vi "test-discretization-14.vi"(8 "error in (no error)":errorcluster) -> (0 "error out":errorcluster, 3 "All Tests Passed":bool)   [LabVIEW 2019]
uses:
  <vilib>/Analysis/Matrix/Datatypes/ComplexMatrix.ctl
  <vilib>/Analysis/Matrix/Datatypes/RealMatrix.ctl
  <vilib>/Analysis/7linalg.llb/Eigenvalue and Vectors Output Option.ctl
  <vilib>/Rock Robotics/WPI/ThirdParty/JAS_Junk/TrajLib/MatBuilder_Create.vi
  <vilib>/Rock Robotics/WPI/ThirdParty/JAS_Junk/TrajLib/MatrixHelper_CoerceSize.vi
  <vilib>/Rock Robotics/WPI/ThirdParty/JAS_Junk/TrajLib/Matrix_Transpose.vi
  <vilib>/Rock Robotics/WPI/ThirdParty/JAS_Junk/TrajLib/Matrix_AssignBlock.vi
  <vilib>/Rock Robotics/WPI/ThirdParty/JAS_Junk/TrajLib/Matrix_Exp.vi
  <vilib>/Rock Robotics/WPI/ThirdParty/JAS_Junk/TrajLib/Matrix_Block.vi
  <vilib>/Analysis/baseanly.llb/A x B.vi
  <vilib>/Analysis/baseanly.llb/Real A x B.vi
  <vilib>/Analysis/7linalg.llb/Transpose Matrix.vi
  <vilib>/Analysis/7linalg.llb/Real Transpose Matrix.vi
  <vilib>/Analysis/_algsub.llb/Matrix Norm.vi
  <vilib>/Analysis/_algsub.llb/Real Matrix Norm.vi
  <vilib>/Analysis/7linalg.llb/Matrix Exp.vi
  <vilib>/Analysis/7linalg.llb/Real Matrix Exp.vi
  <vilib>/Analysis/7linalg.llb/Real Eigenvalues and Vectors.vi
  <vilib>/Analysis/Matrix/Numeric/Multiply/Multiply.vi
  <vilib>/Analysis/Matrix/Numeric/Multiply/Multiply - RM,R.vi
  <vilib>/Analysis/Matrix/Numeric/Add/Add.vi
  <vilib>/Analysis/Matrix/Numeric/Add/Add - RM,RM.vi
  <vilib>/Analysis/Matrix/Numeric/Subtract/Subtract - RM,RM.vi
  <vilib>/Rock Robotics/WPI/ThirdParty/JAS_Junk/TrajLib/Trajectory_Library.lvlib
  <vilib>/Analysis/NI_AALPro.lvlib
  <vilib>/Analysis/Matrix/NI_Matrix.lvlib
panel:
  out "Eigenvalues 2":cdb[](array[numeric])
  out "Pos Semidefiniate 2":bool
  out "error 2":i32
  out "ApproxEquals 2":bool
  out "ApproxEquals":bool
  out "DiscQ Taylor\nNOT":T1
  out "DiscA Taylor\nNOT":T1
  out "Error 2":bool
  out "DiscA":T1
  out "DiscQ Int":T1
  in  "Cluster":cluster{"ContQ":T1, "ContA":T1}
  out "int discq":bool
  out "Pos Semidefiniate":bool
  out "Eigenvectors":T2
  out "error":i32
  out "Eigenvalues":cdb[](array[numeric])
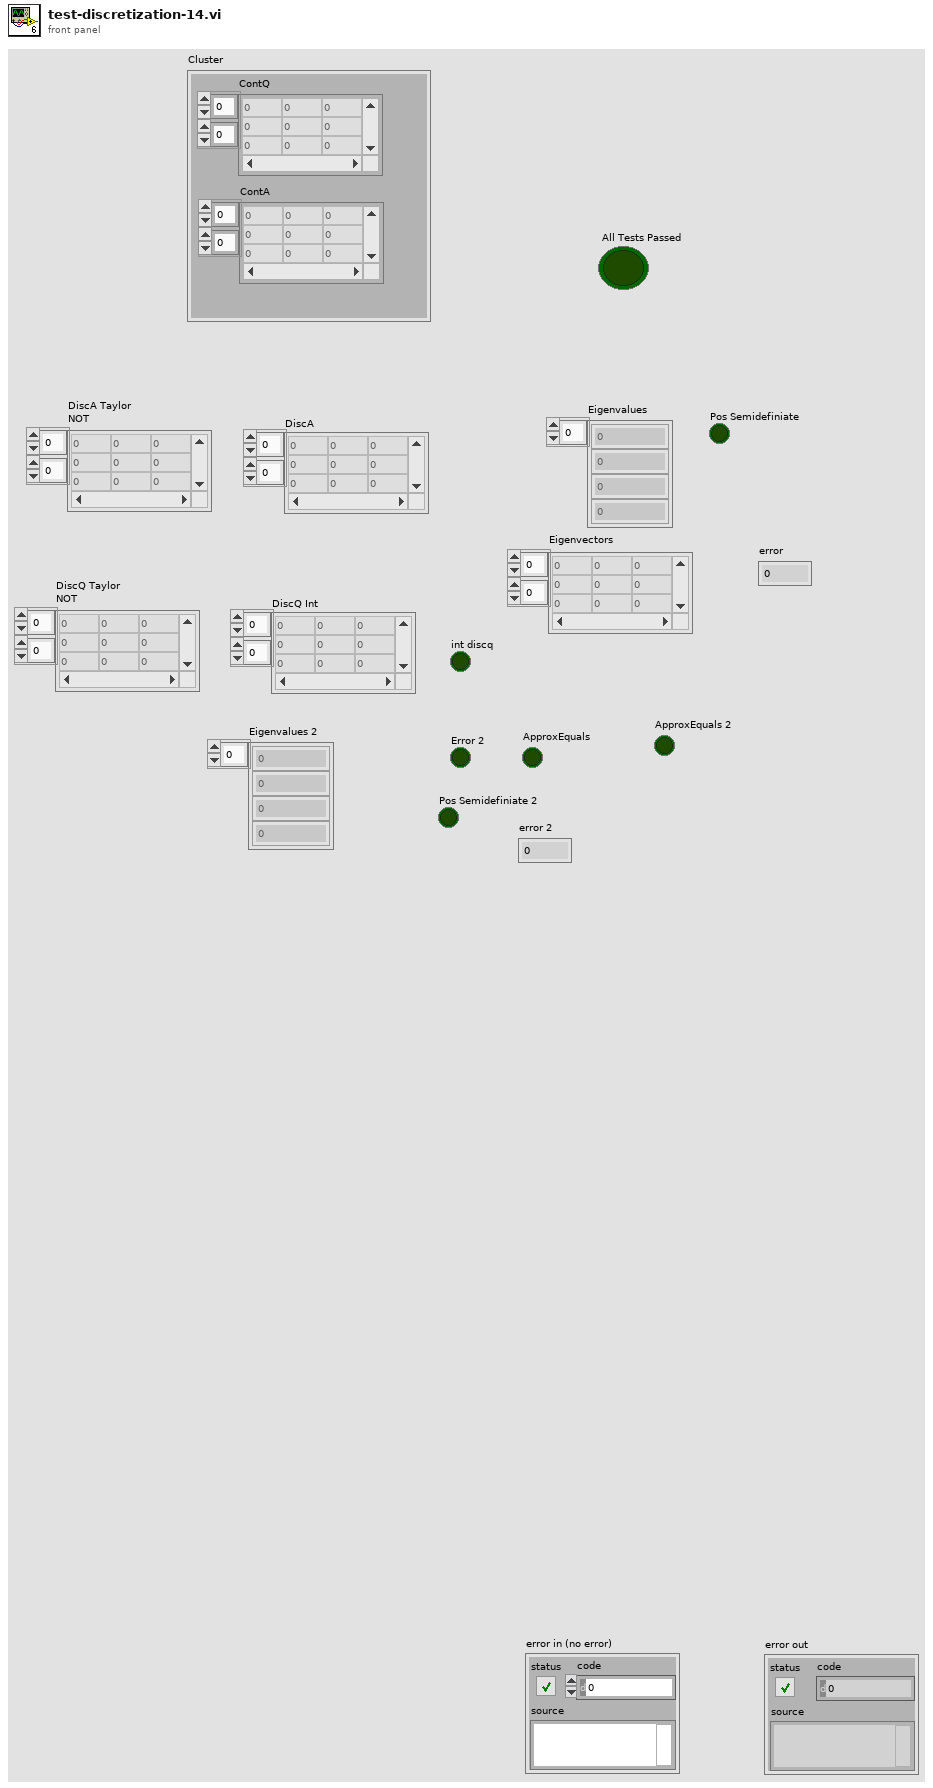
[diagram p1: front panel]
types:
  T1 = typedef "NI_Matrix.lvlib/RealMatrix.ctl" = dbl[][]
  T2 = typedef "NI_Matrix.lvlib/ComplexMatrix.ctl" = cdb[][]
  T3 = typedef "NI_AALPro.lvlib/Eigenvalue and Vectors Output Option.ctl" = i32
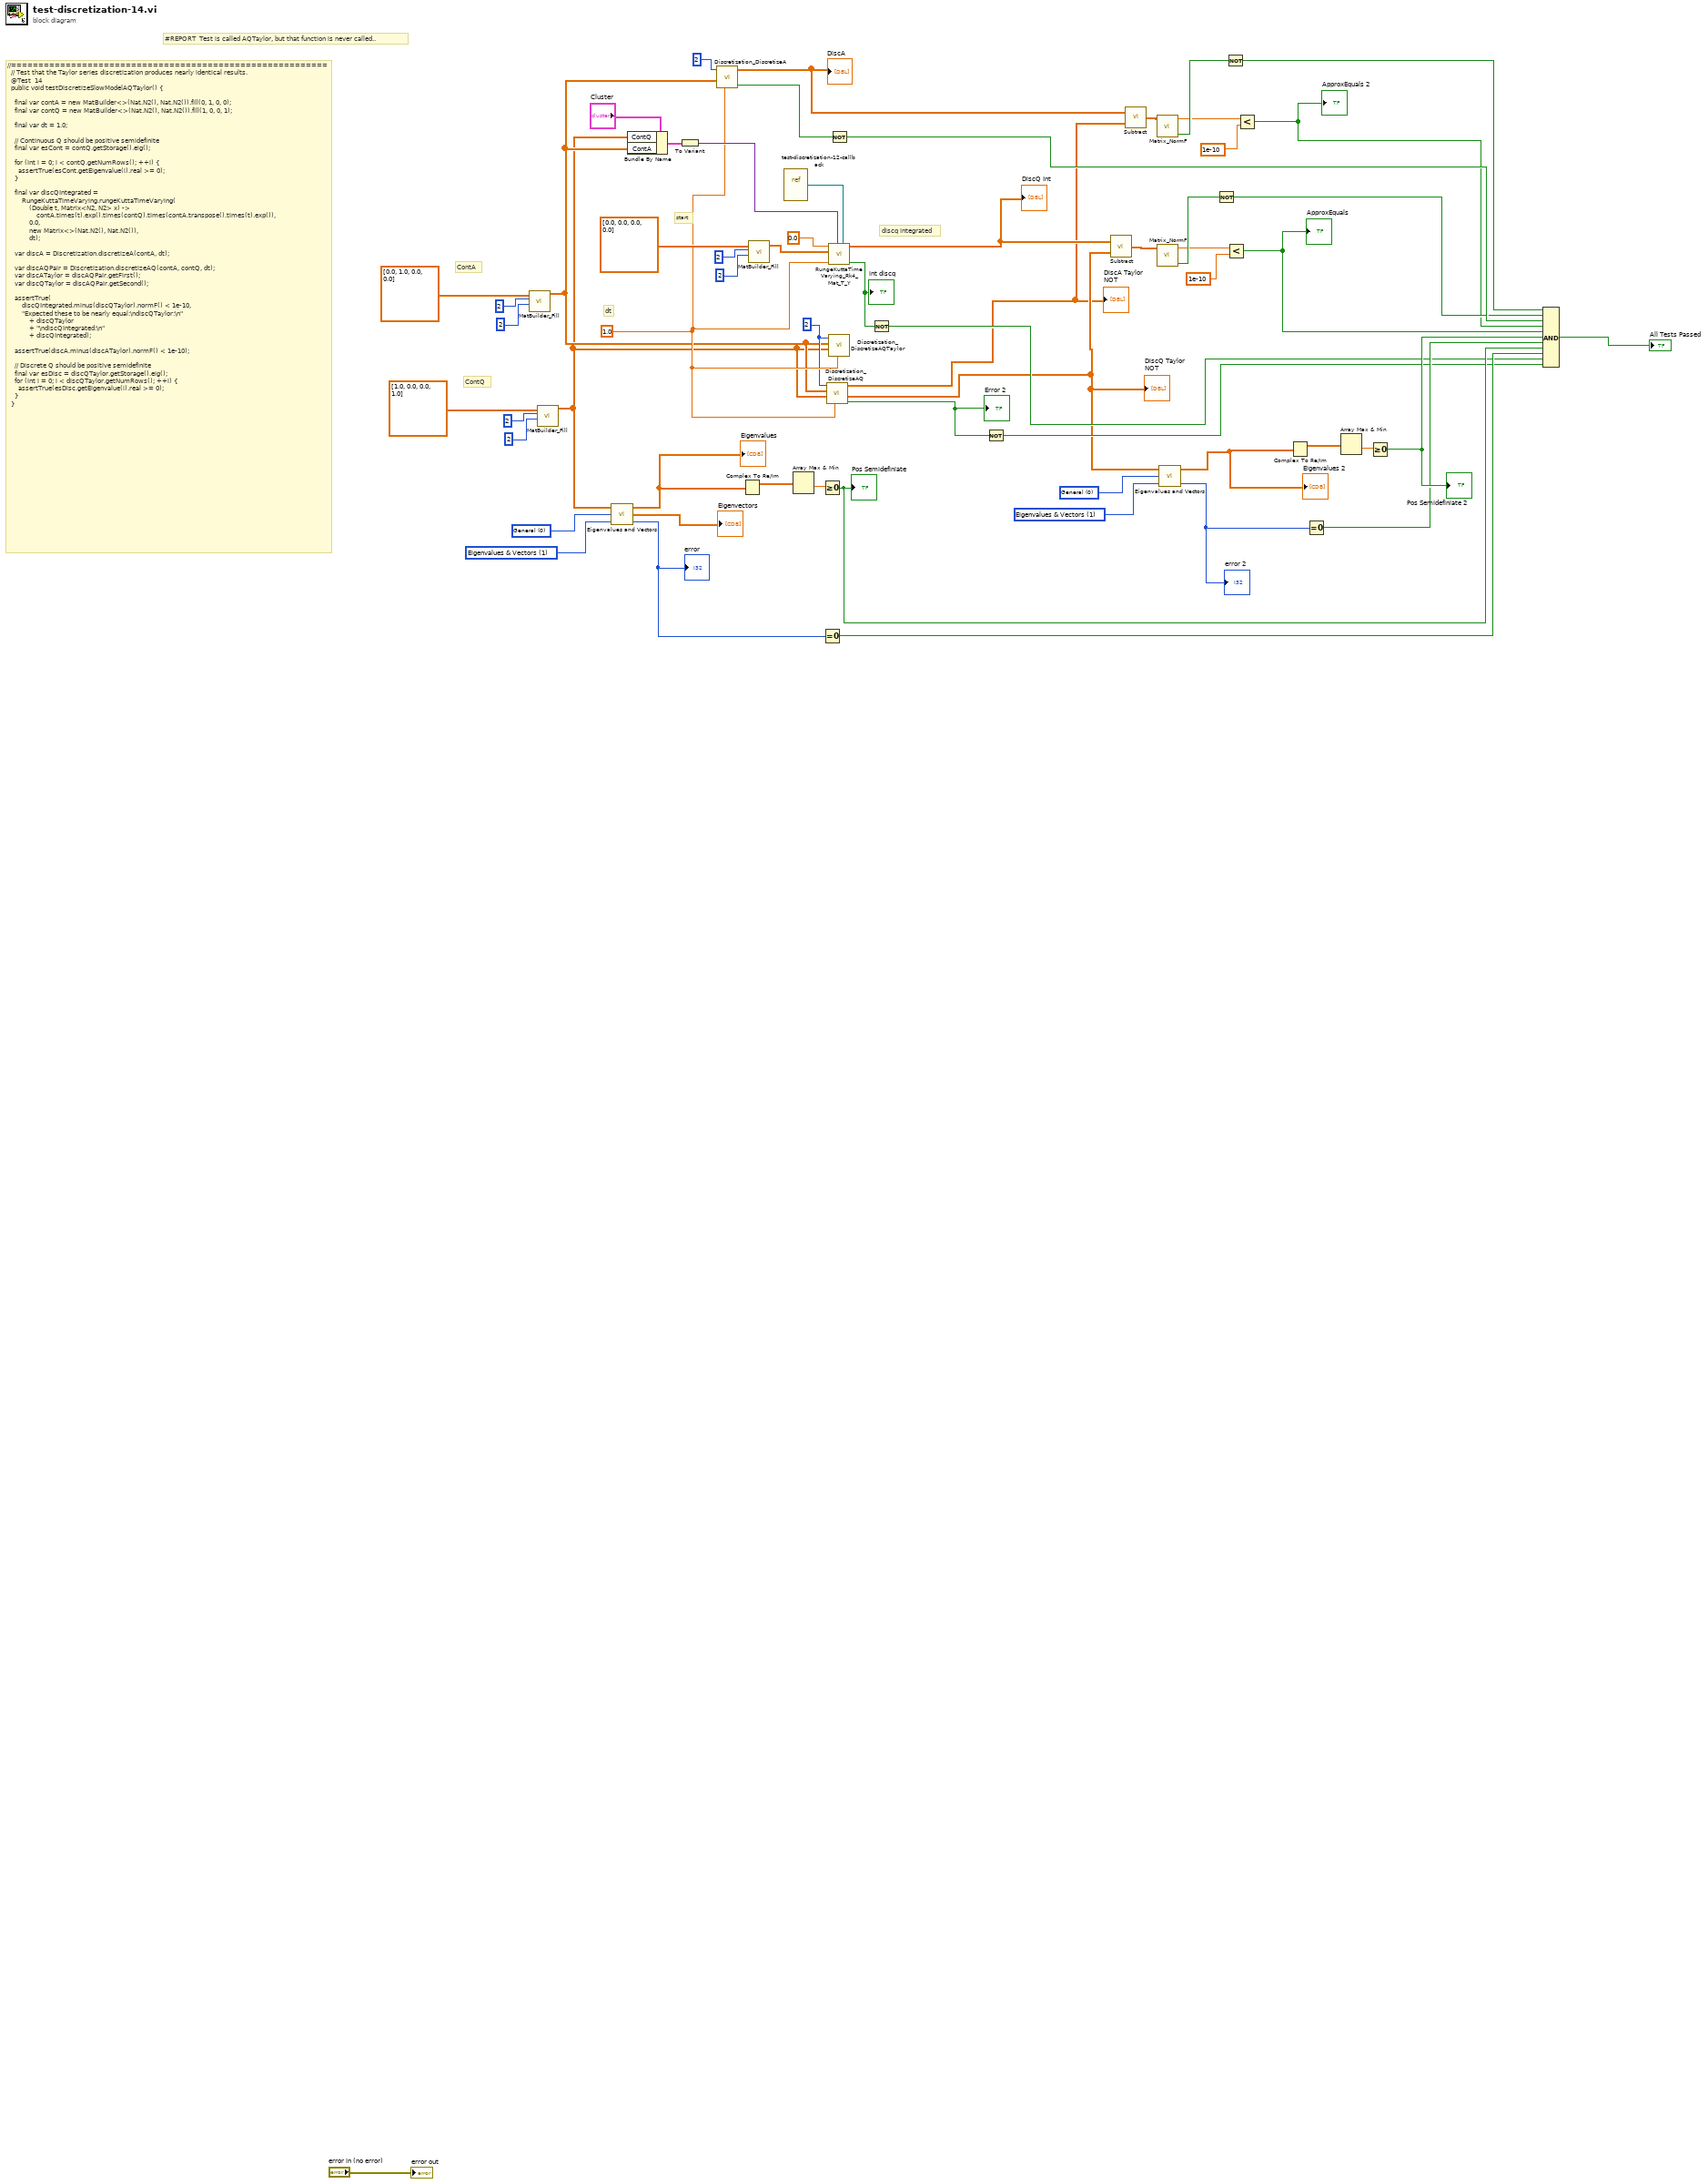
[diagram p0: block diagram]
diagram:
  w27 = T3 1 items=["Eigenvalues", "Eigenvalues & Vectors"] ("output option")
  w28 = 0 items=["General", "Symmetric"] ("matrix type")
  w35 = 2 ("States")
  w36 = 1.0 ("dT_Seconds")
  w53 = T3 1 items=["Eigenvalues", "Eigenvalues & Vectors"] ("output option")
  w54 = 0 items=["General", "Symmetric"] ("matrix type")
  # "#REPORT  Test is called AQTaylor, but that function is never called.."
  # "dt"
  # "discq integrated"
  # "start"
  # "ContQ"
  # "ContA"
  # "//==========================================================\n  // Test that the Taylor series discretization produces nearly identical results.\n  @Test  14\n  public void testDiscretizeSlowModelAQTaylor() {\n\n    final var contA = new MatBuilder<>(Nat.N2(), Nat.N2()).fill(0, 1, 0, 0);\n    final var contQ = new MatBuilder<>(Nat.N2(), Nat.N2()).fill(1, 0, 0, 1);\n\n    final var dt = 1.0;\n\n    // Continuous Q should be positive semidefinite\n    final var esCont = contQ.getStorage().eig();\n\n    for (int i = 0; i < contQ.getNumRows(); ++i) {\n      assertTrue(esCont.getEigenvalue(i).real >= 0);\n    }\n\n    final var discQIntegrated =\n        RungeKuttaTimeVarying.rungeKuttaTimeVarying(\n            (Double t, Matrix<N2, N2> x) ->\n                contA.times(t).exp().times(contQ).times(contA.transpose().times(t).exp()),\n            0.0,\n            new Matrix<>(Nat.N2(), Nat.N2()),\n            dt);\n\n    var discA = Discretization.discretizeA(contA, dt);\n\n    var discAQPair = Discretization.discretizeAQ(contA, contQ, dt);\n    var discATaylor = discAQPair.getFirst();\n    var discQTaylor = discAQPair.getSecond();\n\n    assertTrue(\n        discQIntegrated.minus(discQTaylor).normF() < 1e-10,\n        \"Expected these to be nearly equal:\\ndiscQTaylor:\\n\"\n            + discQTaylor\n            + \"\\ndiscQIntegrated:\\n\"\n            + discQIntegrated);\n\n    assertTrue(discA.minus(discATaylor).normF() < 1e-10);\n\n    // Discrete Q should be positive semidefinite\n    final var esDisc = discQTaylor.getStorage().eig();\n    for (int i = 0; i < discQTaylor.getNumRows(); ++i) {\n      assertTrue(esDisc.getEigenvalue(i).real >= 0);\n    }\n  }"
  n1 = call <vilib>:"MatBuilder_Fill.vi"("Columns"=2, "Rows"=2, "Value List"=dbl[] [0.0, 1.0, 0.0, 0.0]) -> ("output matrix"=w34:T1)  [unwired: 8 in]
  n2 = call <vilib>:"MatBuilder_Fill.vi"("Columns"=2, "Rows"=2, "Value List"=dbl[] [1.0, 0.0, 0.0, 1.0]) -> ("output matrix"=w33:T1)  [unwired: 8 in]
  n3 = call-poly <vilib>:"Eigenvalues and Vectors.vi"("output option"=w53, "matrix type"=w54, "Input Matrix"=w33) -> ("error"=w19:i32, "Eigenvectors"=→"Eigenvectors":T2, "Eigenvalues"=w50:cdb[])
  "Eigenvalues" <- w50
  "error" <- w19
  n4 = Bundle By Name(cluster="Cluster", "ContQ"=w33, "ContA"=w34) -> (w40:cluster{"ContQ":T1, "ContA":T1})
  n5 = To Variant(anything=w40) -> (Variant=w39:variant)
  n6 = call <vilib>:"Discretization_DiscretizeA.vi"("dT_Seconds"=w36, "ContA"=w34, "States"=2) -> ("Error"=w15:bool, "DiscA"=w29:T1)  [unwired: 7 in]
  "DiscA" <- w29
  n7 = Complex To Re/Im(x + iy=w50) -> (x=w49:dbl[])  [unwired: 1 out]
  n8 = call <vilib>:"MatBuilder_Fill.vi"("Columns"=2, "Rows"=2, "Value List"=dbl[] [0.0, 0.0, 0.0, 0.0]) -> ("output matrix"=w42:T1)  [unwired: 8 in]
  n9 = vi-ref "test-discretization-12-callback.vi"() -> (w47:refnum<vi>)
  n10 = Array Max & Min(array=w49) -> (min value=w48:dbl)  [unwired: 3 out]
  n11 = Greater Or Equal To 0?(x=w48) -> (x >= 0?=w20:bool)
  "Pos Semidefiniate" <- w20
  n12 = Equal To 0?(x=w19) -> (x = 0?=w18:bool)
  n13 = call <vilib>:"Discretization_DiscretizeAQ.vi"("dT_Seconds"=w36, "ContQ"=w33, "ContA"=w34, "States"=w35) -> ("Error"=w9:bool, "DiscQ"=w8:T1, "DiscA"=w7:T1)  [unwired: 5 in]
  "Error 2" <- w9
  "DiscA Taylor\nNOT" <- w7
  "DiscQ Taylor\nNOT" <- w8
  n14 = Not(x=w15) -> (.not. x?=w14:bool)
  n15 = call <vilib>:"RungeKuttaTimeVarying_Rk4_Mat_T_Y.vi"("Func_T_Y_Extra"=w47, "PassedData"=w39, "dT_Seconds"=w36, "Y"=w42, "T"=0.0) -> ("Error"=w38:bool, "OUTPUT"=w32:T1)  [unwired: 5 in]
  "int discq" <- w38
  "DiscQ Int" <- w32
  n16 = call <vilib>:"Discretization_DiscretizeAQTaylor.vi"("dT_Seconds"=w36, "ContQ"=w33, "ContA"=w34, "States"=w35) -> ()  [unwired: 5 in, 3 out]
  n17 = Not(x=w38) -> (.not. x?=w16:bool)
  n18 = Not(x=w9) -> (.not. x?=w17:bool)
  n19 = call-poly <vilib>:"Subtract.vi"("Real Matrix B"=w8, "Real Matrix A"=w32) -> ("A - B"=w31:T1)
  n20 = call-poly <vilib>:"Subtract.vi"("Real Matrix B"=w7, "Real Matrix A"=w29) -> ("A - B"=w30:T1)
  n21 = call <vilib>:"Matrix_NormF.vi"("input matrix"=w30) -> ("Error"=w13:bool, "normF"=w3:dbl)  [unwired: 9 in]
  n22 = call <vilib>:"Matrix_NormF.vi"("input matrix"=w31) -> ("Error"=w12:bool, "normF"=w6:dbl)  [unwired: 9 in]
  n23 = call-poly <vilib>:"Eigenvalues and Vectors.vi"("output option"=w27, "matrix type"=w28, "Input Matrix"=w8) -> ("error"=w22:i32, "Eigenvalues"=w26:cdb[])  [unwired: 1 out]
  "error 2" <- w22
  "Eigenvalues 2" <- w26
  n24 = Not(x=w12) -> (.not. x?=w11:bool)
  n25 = Not(x=w13) -> (.not. x?=w10:bool)
  n26 = Less?(x=w6, y=1e-10 ("Tolerance")) -> (x < y?=w4:bool)
  "ApproxEquals" <- w4
  n27 = Less?(x=w3, y=1e-10 ("Tolerance")) -> (x < y?=w1:bool)
  "ApproxEquals 2" <- w1
  n28 = Complex To Re/Im(x + iy=w26) -> (x=w25:dbl[])  [unwired: 1 out]
  n29 = Equal To 0?(x=w22) -> (x = 0?=w21:bool)
  n30 = Array Max & Min(array=w25) -> (min value=w24:dbl)  [unwired: 3 out]
  n31 = Greater Or Equal To 0?(x=w24) -> (x >= 0?=w23:bool)
  "Pos Semidefiniate 2" <- w23
  n32 = Compound Arithmetic op=AND(w10, w11, w14, w1, w4, w23, w21, w20, w18, w16, w17) -> (→"All Tests Passed":bool)
  "error out" <- "error in (no error)"
